vi "fun_Points2TimeLength.vi"(10 "HDAWG Sample Rate (2.4GSa/s)":dbl=2400000000.0 format="%#_13p", 11 "Points in AWG":dbl) -> (3 "Time Length (s)":dbl format="%#_6ps")   [LabVIEW 2016]
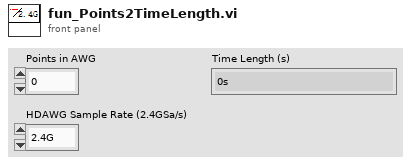
[diagram p1: front panel]
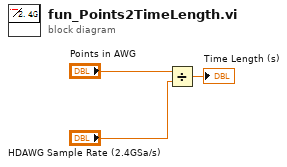
[diagram p0: block diagram]
diagram:
  n1 = Divide(x="Points in AWG", y="HDAWG Sample Rate (2.4GSa/s)") -> (x/y=→"Time Length (s)":dbl)
